vi "PeakDetect.vi"(11 "Data":u16[](array[numeric])) -> (0 "Minimum (Index)":u8, 1 "Minimum (Value)":u16, 2 "Maximum (Index)":u8, 3 "Maximum (Value)":u16)   [LabVIEW 2013]
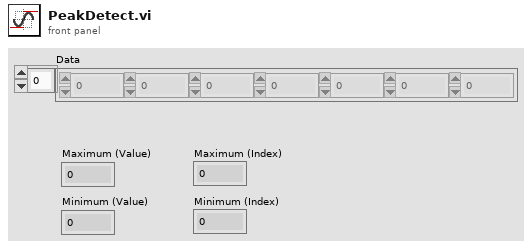
[diagram p1: front panel]
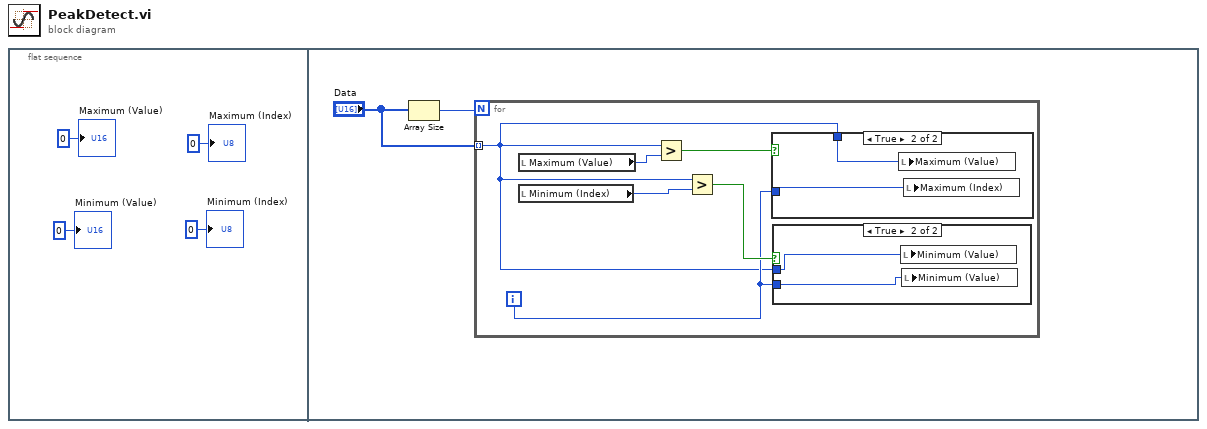
[diagram p0: block diagram]
diagram:
  n1 = flat-sequence {
    frame #0 {
      "Maximum (Value)" <- u16 0 ("Maximum (Value)")
      "Maximum (Index)" <- u8 0 ("Maximum (Index)")
      "Minimum (Value)" <- u16 0 ("Minimum (Value)")
      "Minimum (Index)" <- u8 0 ("Minimum (Index)")
    }
    frame #1 {
      n2 = Array Size(array="Data") -> (size(s)=w6:i32)
      n3 = for {
        N: w6 -> [_]
        tunnel: "Data" -> [w7] mode=indexing
        i -> [w8]
        n4 = local read "Maximum (Value)"() -> (w12:u16)
        n5 = local read "Minimum (Index)"() -> (w11:u8)
        n6 = Greater?(x=w7, y=w12) -> (0:w10:bool)
        n7 = Greater?(x=w7, y=w11) -> (0:w9:bool)
        n8 = case shown="True" w10 {
          tunnel: w7 -> [_ w16]
          tunnel: w8 -> [_ w15]
          frame False {
          }
          frame True {
            n9 = local write "Maximum (Value)"(w16) -> ()
            n10 = local write "Maximum (Index)"(w15) -> ()
          }
        }
        n11 = case shown="True" w9 {
          tunnel: w7 -> [_ w14]
          tunnel: w8 -> [_ w13]
          frame False {
          }
          frame True {
            n12 = local write "Minimum (Value)"(w14) -> ()
            n13 = local write "Minimum (Value)"(w13) -> ()
          }
        }
      }
    }
  }
